vi "merge_x_y.vi"(9 "frekans size":i32, 10 "y1_y2":dbl[][](array[numeric]), 11 "x1_x2":dbl[][](array[numeric])) -> (3 "x1_x2_y1_y2":dbl[][](array[numeric]))   [LabVIEW 2014]
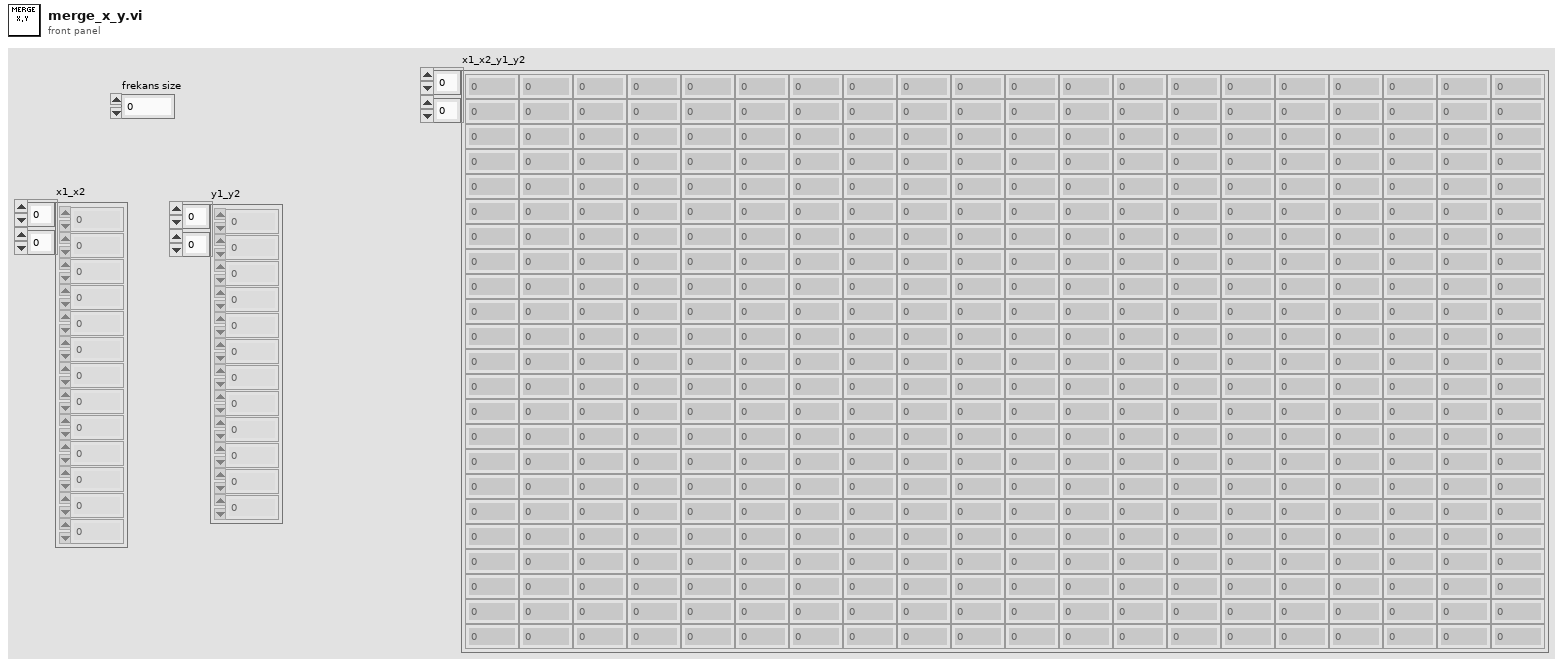
[diagram p1: front panel]
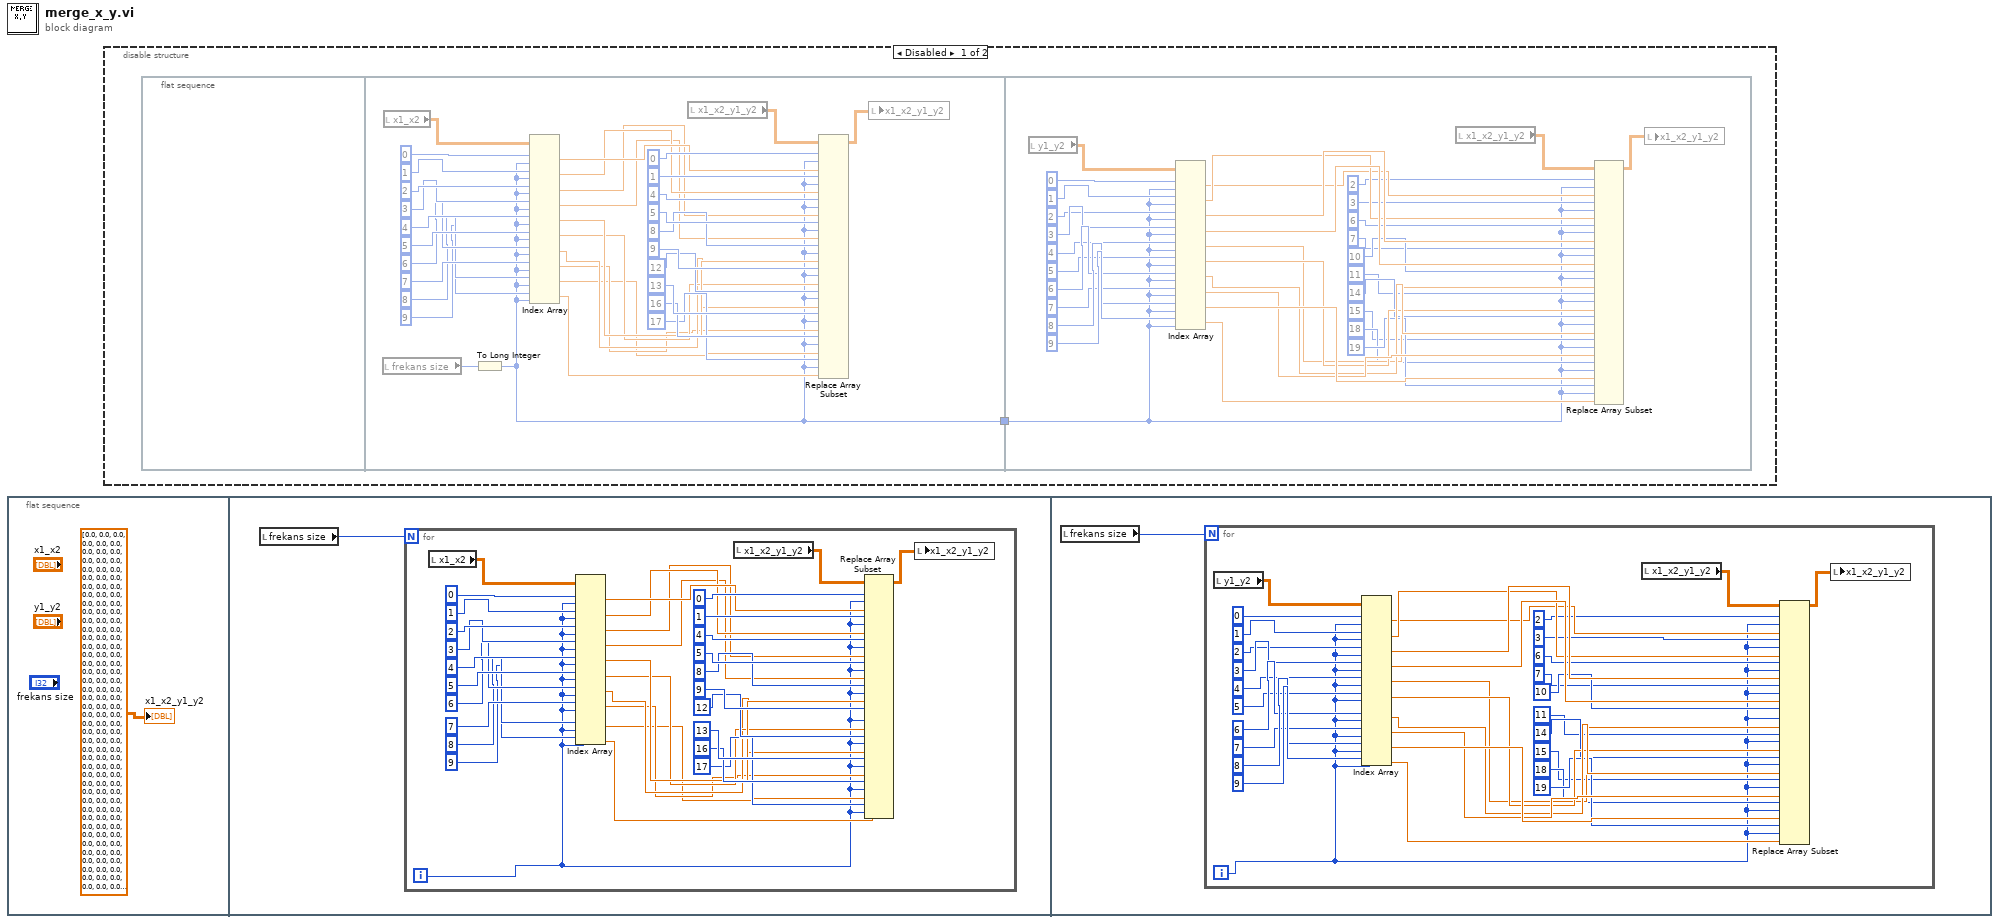
[diagram p0: block diagram]
diagram:
  n1 = flat-sequence {
    frame #0 {
      "x1_x2_y1_y2" <- dbl[][] [[0.0, 0.0, 0.0, 0.0, 0.0, 0.0, 0.0, 0.0, 0.0, 0.0, 0.0, 0.0, 0.0, 0.0, 0.0, 0.0, 0.0, 0.0, 0.0, 0.0], [0.0, 0.0, 0.0, 0.0, 0.0, 0.0, 0.0, 0.0, 0.0, 0.0, 0.0, 0.0, 0.0, 0.0, 0.0, 0.0, 0.0, 0.0, 0.0, 0.0], [0.0, 0.0, 0.0, 0.0, 0.0, 0.0, 0.0, 0.0, 0.0, 0.0, 0.0, 0.0, 0.0, 0.0, 0.0, 0.0, 0.0, 0.0, 0.0, 0.0], [0.0, 0.0, 0.0, 0.0, 0.0, 0.0, 0.0, 0.0, 0.0, 0.0, 0.0, 0.0, 0.0, 0.0, 0.0, 0.0, 0.0, 0.0, 0.0, 0.0], [0.0, 0.0, 0.0, 0.0, 0.0, 0.0, 0.0, 0.0, 0.0, 0.0, 0.0, 0.0, 0.0, 0.0, 0.0, 0.0, 0.0, 0.0, 0.0, 0.0], [0.0, 0.0, 0.0, 0.0, 0.0, 0.0, 0.0, 0.0, 0.0, 0.0, 0.0, 0.0, 0.0, 0.0, 0.0, 0.0, 0.0, 0.0, 0.0, 0.0], [0.0, 0.0, 0.0, 0.0, 0.0, 0.0, 0.0, 0.0, 0.0, 0.0, 0.0, 0.0, 0.0, 0.0, 0.0, 0.0, 0.0, 0.0, 0.0, 0.0], [0.0, 0.0, 0.0, 0.0, 0.0, 0.0, 0.0, 0.0, 0.0, 0.0, 0.0, 0.0, 0.0, 0.0, 0.0, 0.0, 0.0, 0.0, 0.0, 0.0], [0.0, 0.0, 0.0, 0.0, 0.0, 0.0, 0.0, 0.0, 0.0, 0.0, 0.0, 0.0, 0.0, 0.0, 0.0, 0.0, 0.0, 0.0, 0.0, 0.0], [0.0, 0.0, 0.0, 0.0, 0.0, 0.0, 0.0, 0.0, 0.0, 0.0, 0.0, 0.0, 0.0, 0.0, 0.0, 0.0, 0.0, 0.0, 0.0, 0.0], [0.0, 0.0, 0.0, 0.0, 0.0, 0.0, 0.0, 0.0, 0.0, 0.0, 0.0, 0.0, 0.0, 0.0, 0.0, 0.0, 0.0, 0.0, 0.0, 0.0], [0.0, 0.0, 0.0, 0.0, 0.0, 0.0, 0.0, 0.0, 0.0, 0.0, 0.0, 0.0, 0.0, 0.0, 0.0, 0.0, 0.0, 0.0, 0.0, 0.0], [0.0, 0.0, 0.0, 0.0, 0.0, 0.0, 0.0, 0.0, 0.0, 0.0, 0.0, 0.0, 0.0, 0.0, 0.0, 0.0, 0.0, 0.0, 0.0, 0.0], [0.0, 0.0, 0.0, 0.0, 0.0, 0.0, 0.0, 0.0, 0.0, 0.0, 0.0, 0.0, 0.0, 0.0, 0.0, 0.0, 0.0, 0.0, 0.0, 0.0], [0.0, 0.0, 0.0, 0.0, 0.0, 0.0, 0.0, 0.0, 0.0, 0.0, 0.0, 0.0, 0.0, 0.0, 0.0, 0.0, 0.0, 0.0, 0.0, 0.0], [0.0, 0.0, 0.0, 0.0, 0.0, 0.0, 0.0, 0.0, 0.0, 0.0, 0.0, 0.0, 0.0, 0.0, 0.0, 0.0, 0.0, 0.0, 0.0, 0.0], [0.0, 0.0, 0.0, 0.0, 0.0, 0.0, 0.0, 0.0, 0.0, 0.0, 0.0, 0.0, 0.0, 0.0, 0.0, 0.0, 0.0, 0.0, 0.0, 0.0], [0.0, 0.0, 0.0, 0.0, 0.0, 0.0, 0.0, 0.0, 0.0, 0.0, 0.0, 0.0, 0.0, 0.0, 0.0, 0.0, 0.0, 0.0, 0.0, 0.0], [0.0, 0.0, 0.0, 0.0, 0.0, 0.0, 0.0, 0.0, 0.0, 0.0, 0.0, 0.0, 0.0, 0.0, 0.0, 0.0, 0.0, 0.0, 0.0, 0.0], [0.0, 0.0, 0.0, 0.0, 0.0, 0.0, 0.0, 0.0, 0.0, 0.0, 0.0, 0.0, 0.0, 0.0, 0.0, 0.0, 0.0, 0.0, 0.0, 0.0]] ("x1_x2_y1_y2")
    }
    frame #1 {
      n2 = local read "frekans size"() -> (w2:i32)
      n3 = for {
        N: w2 -> [_]
        i -> [w3]
        n4 = local read "x1_x2"() -> (w24:dbl[][])
        n5 = Index Array(array=w24, index (row) #1=0, index (col) #1=w3, index (row) #2=1, index (col) #2=w3, index (row) #3=2, index (col) #3=w3, index (row) #4=3, index (col) #4=w3, index (row) #5=4, index (col) #5=w3, index (row) #6=5, index (col) #6=w3, index (row) #7=6, index (col) #7=w3, index (row) #8=7, index (col) #8=w3, index (row) #9=8, index (col) #9=w3, index (row) #10=9, index (col) #10=w3) -> (element #1=w13:dbl, element #2=w12:dbl, element #3=w11:dbl, element #4=w10:dbl, element #5=w9:dbl, element #6=w8:dbl, element #7=w7:dbl, element #8=w6:dbl, element #9=w5:dbl, element #10=w4:dbl)
        n6 = local read "x1_x2_y1_y2"() -> (w36:dbl[][])
        n7 = Replace Array Subset(array=w36, new element #1=w13, index (row) #1=0, index (col) #1=w3, new element #2=w12, index (row) #2=1, index (col) #2=w3, new element #3=w11, index (row) #3=4, index (col) #3=w3, new element #4=w10, index (row) #4=5, index (col) #4=w3, new element #5=w9, index (row) #5=8, index (col) #5=w3, new element #6=w8, index (row) #6=9, index (col) #6=w3, new element #7=w7, index (row) #7=12, index (col) #7=w3, new element #8=w6, index (row) #8=13, index (col) #8=w3, new element #9=w5, index (row) #9=16, index (col) #9=w3, new element #10=w4, index (row) #10=17, index (col) #10=w3) -> (w35:dbl[][])
        n8 = local write "x1_x2_y1_y2"(w35) -> ()
      }
    }
    frame #2 {
      n9 = local read "frekans size"() -> (w37:i32)
      n10 = for {
        N: w37 -> [_]
        i -> [w38]
        n11 = local read "y1_y2"() -> (w51:dbl[][])
        n12 = Index Array(array=w51, index (row) #1=0, index (col) #1=w38, index (row) #2=1, index (col) #2=w38, index (row) #3=2, index (col) #3=w38, index (row) #4=3, index (col) #4=w38, index (row) #5=4, index (col) #5=w38, index (row) #6=5, index (col) #6=w38, index (row) #7=6, index (col) #7=w38, index (row) #8=7, index (col) #8=w38, index (row) #9=8, index (col) #9=w38, index (row) #10=9, index (col) #10=w38) -> (element #1=w62:dbl, element #2=w63:dbl, element #3=w64:dbl, element #4=w65:dbl, element #5=w66:dbl, element #6=w67:dbl, element #7=w68:dbl, element #8=w69:dbl, element #9=w70:dbl, element #10=w71:dbl)
        n13 = local read "x1_x2_y1_y2"() -> (w39:dbl[][])
        n14 = Replace Array Subset(array=w39, new element #1=w62, index (row) #1=2, index (col) #1=w38, new element #2=w63, index (row) #2=3, index (col) #2=w38, new element #3=w64, index (row) #3=6, index (col) #3=w38, new element #4=w65, index (row) #4=7, index (col) #4=w38, new element #5=w66, index (row) #5=10, index (col) #5=w38, new element #6=w67, index (row) #6=11, index (col) #6=w38, new element #7=w68, index (row) #7=14, index (col) #7=w38, new element #8=w69, index (row) #8=15, index (col) #8=w38, new element #9=w70, index (row) #9=18, index (col) #9=w38, new element #10=w71, index (row) #10=19, index (col) #10=w38) -> (w40:dbl[][])
        n15 = local write "x1_x2_y1_y2"(w40) -> ()
      }
    }
  }
  n16 = disable-structure shown="Disabled" {
    frame Disabled {
      n17 = flat-sequence {
        tunnel: [w73] -> w72
        tunnel: w72 -> [w108]
        frame #0 {
        }
        frame #1 {
          n18 = local read "frekans size"() -> (w74:i32)
          n19 = local read "x1_x2"() -> (w95:dbl[][])
          n20 = To Long Integer(number=w74) -> (32bit integer=w73:i32)
          n21 = Index Array(array=w95, index (row) #1=0, index (col) #1=w73, index (row) #2=1, index (col) #2=w73, index (row) #3=2, index (col) #3=w73, index (row) #4=3, index (col) #4=w73, index (row) #5=4, index (col) #5=w73, index (row) #6=5, index (col) #6=w73, index (row) #7=6, index (col) #7=w73, index (row) #8=7, index (col) #8=w73, index (row) #9=8, index (col) #9=w73, index (row) #10=9, index (col) #10=w73) -> (element #1=w84:dbl, element #2=w83:dbl, element #3=w82:dbl, element #4=w81:dbl, element #5=w80:dbl, element #6=w79:dbl, element #7=w78:dbl, element #8=w77:dbl, element #9=w76:dbl, element #10=w75:dbl)
          n22 = local read "x1_x2_y1_y2"() -> (w107:dbl[][])
          n23 = Replace Array Subset(array=w107, new element #1=w84, index (row) #1=0, index (col) #1=w73, new element #2=w83, index (row) #2=1, index (col) #2=w73, new element #3=w82, index (row) #3=4, index (col) #3=w73, new element #4=w81, index (row) #4=5, index (col) #4=w73, new element #5=w80, index (row) #5=8, index (col) #5=w73, new element #6=w79, index (row) #6=9, index (col) #6=w73, new element #7=w78, index (row) #7=12, index (col) #7=w73, new element #8=w77, index (row) #8=13, index (col) #8=w73, new element #9=w76, index (row) #9=16, index (col) #9=w73, new element #10=w75, index (row) #10=17, index (col) #10=w73) -> (w106:dbl[][])
          n24 = local write "x1_x2_y1_y2"(w106) -> ()
        }
        frame #2 {
          n25 = local read "y1_y2"() -> (w121:dbl[][])
          n26 = Index Array(array=w121, index (row) #1=0, index (col) #1=w108, index (row) #2=1, index (col) #2=w108, index (row) #3=2, index (col) #3=w108, index (row) #4=3, index (col) #4=w108, index (row) #5=4, index (col) #5=w108, index (row) #6=5, index (col) #6=w108, index (row) #7=6, index (col) #7=w108, index (row) #8=7, index (col) #8=w108, index (row) #9=8, index (col) #9=w108, index (row) #10=9, index (col) #10=w108) -> (element #1=w132:dbl, element #2=w133:dbl, element #3=w134:dbl, element #4=w135:dbl, element #5=w136:dbl, element #6=w137:dbl, element #7=w138:dbl, element #8=w139:dbl, element #9=w140:dbl, element #10=w141:dbl)
          n27 = local read "x1_x2_y1_y2"() -> (w109:dbl[][])
          n28 = Replace Array Subset(array=w109, new element #1=w132, index (row) #1=2, index (col) #1=w108, new element #2=w133, index (row) #2=3, index (col) #2=w108, new element #3=w134, index (row) #3=6, index (col) #3=w108, new element #4=w135, index (row) #4=7, index (col) #4=w108, new element #5=w136, index (row) #5=10, index (col) #5=w108, new element #6=w137, index (row) #6=11, index (col) #6=w108, new element #7=w138, index (row) #7=14, index (col) #7=w108, new element #8=w139, index (row) #8=15, index (col) #8=w108, new element #9=w140, index (row) #9=18, index (col) #9=w108, new element #10=w141, index (row) #10=19, index (col) #10=w108) -> (w110:dbl[][])
          n29 = local write "x1_x2_y1_y2"(w110) -> ()
        }
      }
    }
    frame Enabled {
    }
  }
